vi "Review File.vi"(6 "Row Index":i32, 8 "error in":errorcluster, 11 "Peer Review in":refnum<class "Peer Review.lvclass">) -> (0 "error out":errorcluster, 3 "Peer Review out":refnum<class "Peer Review.lvclass">)   [LabVIEW 2020, in "Peer Review.lvclass"]
uses:
  Peer Review.lvclass
  Peer Review.lvclass/Peer Review.ctl
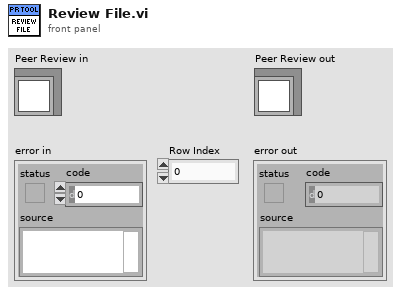
[diagram p1: front panel]
types:
  T1 = typedef "Peer Review.lvclass/File Info.ctl" = cluster{"File ID":i32, "Commit ID":i32, "Reviewed Hash":string, "Relative Path":string, "File Path":path, "File Checksum":string, "State":T2, "FP Changes":i32, "BD Changes":i32, "FP Bounds Error":dbl, "BD Bounds Error":dbl, "Lines Added":i32, "Lines Removed":i32, "Analysis Passes":i32, "Analysis Fails":i32, "Attribute Changes":i32, "Reentrancy State":string, "Cyclomatic Complexity":i32, "Node Count":i32, "Revision Number":u32, "LabVIEW Version":string, "Description":string, "Master Path":path, "Master Checksum":string, "VI Type":T3, "LabVIEW File":bool, "Review Complete":bool, "File Ref":refnum<vi>, "Master Revision":u32}
  T2 = typedef "Peer Review.lvclass/File State.ctl" = enum16{"Interrogation Needed", "Modified", "Deleted", "Added", "Matches Previous", "No Changes", "Moved", "Empty File"}
  T3 = typedef "Peer Review.lvclass/VI Type.ctl" = enum32{"invalid VI type", "Standard VI", "Control VI", "Global VI", "Polymorphic VI", "Configuration VI", "SubSystem", "Facade VI", "Method VI", "Statechart Diagram VI"}
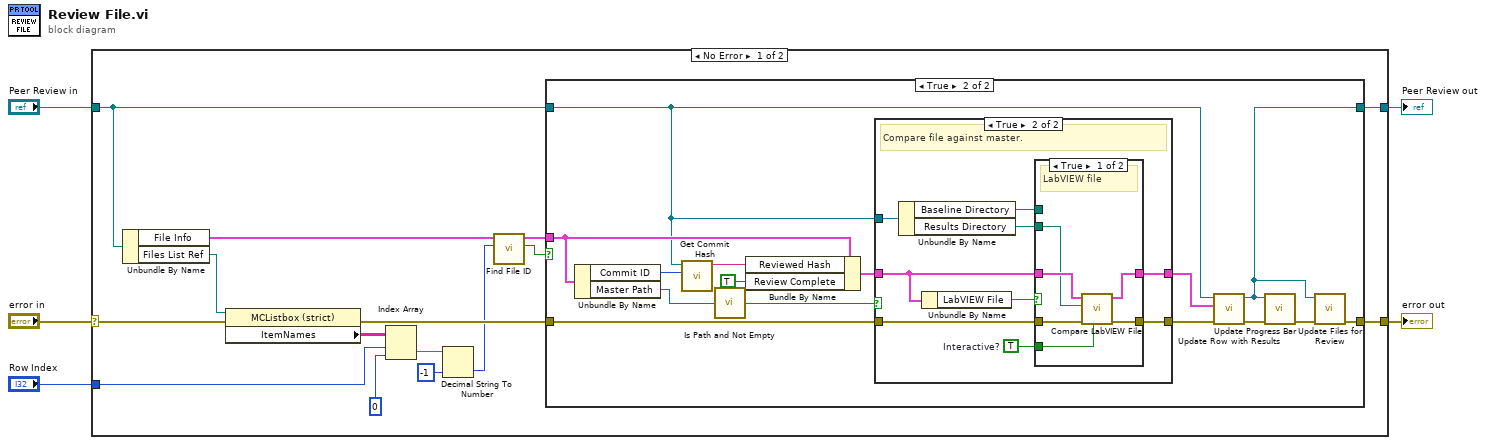
[diagram p0: block diagram]
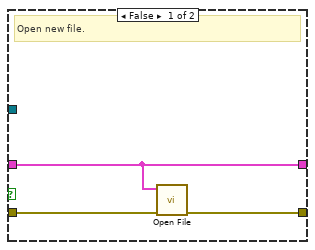
[diagram p3: hidden frame]
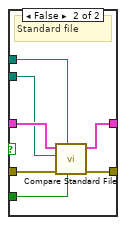
[diagram p4: hidden frame]
diagram:
  n1 = case shown="No Error" "error in" {
    selector: "error in" -> [w15 w64]
    tunnel: "Peer Review in" -> [w20 w63]
    tunnel: [w19 w64] -> w3
    tunnel: "Row Index" -> [w13 _]
    tunnel: [w18 w63] -> w1
    frame No Error {
      n2 = Unbundle By Name(w20) -> ("File Info"=w9:T1[], "Files List Ref"=w12:refnum<vi>)
      n3 = property on="Property Node" class="MCListbox (strict)"(reference=w12, error in=w15) -> (error out=w14:errorcluster, "ItemNames"=w17:string[][])  [unwired: 1 out]
      n4 = Index Array(array=w17, index (row)=w13, index (col)=0 ("disabled index (col)")) -> (element=w16:string)
      n5 = Decimal String To Number(string=w16, default (0L)=-1 ("default (0 I32)")) -> (number=w8:i32)  [unwired: 1 in, 1 out]
      n6 = call "Find File ID.vi"("File ID"=w8, "File List"=w9) -> ("Found?"=w6:bool, "File Info"=w7:T1)  [unwired: 7 in, 1 out]
      n7 = case shown="True" w6 {
        tunnel: w20 -> [w22 w27]
        tunnel: [w21 w24] -> w19
        tunnel: [w22 w23] -> w18
        tunnel: w14 -> [w21 w30]
        tunnel: w7 -> [_ w37]
        frame False {
        }
        frame True {
          n8 = Unbundle By Name(w37) -> ("Commit ID"=w36:i32, "Master Path"=w31:path)
          n9 = call "Get Commit Hash.vi"("Commit ID"=w36, "Peer Review"=w27) -> ("Hash"=w35:string)  [unwired: 9 in]
          n10 = call <vilib>:"Is Path and Not Empty.vi"("path"=w31) -> ("Is Path and Not Empty?"=w33:bool)  [unwired: 4 in]
          n11 = Bundle By Name(cluster=w37, "Reviewed Hash"=w35, "Review Complete"=TRUE) -> (w32:T1)
          n12 = case shown="True" w33 {
            tunnel: w30 -> [w40 w48]
            tunnel: [w38 w47] -> w29
            tunnel: w27 -> [_ w45]
            tunnel: w32 -> [w39 w42]
            tunnel: [w39 w46] -> w28
            frame False {
              # "Open new file."
              n13 = call "Open File.vi"("error in"=w40, "File Info"=w39) -> ("error out"=w38:errorcluster)  [unwired: 9 in]
            }
            frame True {
              w49 = TRUE  # Interactive?
              # "Compare file against master."
              n14 = Unbundle By Name(w45) -> ("Baseline Directory"=w43:path, "Results Directory"=w44:path)
              n15 = Unbundle By Name(w42) -> ("LabVIEW File"=w41:bool)
              n16 = case shown="True" w41 {
                tunnel: w48 -> [w55 w62]
                tunnel: [w54 w61] -> w47
                tunnel: [w53 w60] -> w46
                tunnel: w49 -> [w50 w58]
                tunnel: w42 -> [w52 w59]
                tunnel: w44 -> [w51 w57]
                tunnel: w43 -> [_ w56]
                frame True {
                  # "LabVIEW file"
                  n17 = call "Compare LabVIEW File.vi"("Interactive?"=w50, "error in"=w55, "Results Directory"=w51, "File Info in"=w52) -> ("error out"=w54:errorcluster, "File Info out"=w53:T1)  [unwired: 6 in]
                }
                frame False {
                  # "Standard file"
                  n18 = call "Compare Standard File.vi"("Interactive?"=w58, "Baseline Directory"=w56, "error in"=w62, "Results Directory"=w57, "File Info in"=w59) -> ("error out"=w61:errorcluster, "File Info out"=w60:T1)  [unwired: 5 in]
                }
              }
            }
          }
          n19 = call "Update Row with Results.vi"("error in"=w29, "File Info"=w28, "Peer Review in"=w27) -> ("error out"=w26:errorcluster, "Peer Review out"=w23:refnum<class "Peer Review.lvclass">)  [unwired: 7 in]
          n20 = call "Update Progress Bar.vi"("error in"=w26, "Peer Review"=w23) -> ("error out"=w25:errorcluster)  [unwired: 9 in]
          n21 = call "Update Files for Review.vi"("error in"=w25, "Peer Review"=w23) -> ("error out"=w24:errorcluster)  [unwired: 9 in]
        }
      }
    }
    frame Error {
    }
  }
  "error out" <- w3
  "Peer Review out" <- w1
